vi "GenerateWaveform.vi"(5 "FPGA Cycle Parameters XY":T4={"FPGA Cycle Parameters X"={"Imaging cycles"=285714, "Settling cycles"=71429, "Resting cycles"=42857, "Phase advance per cycle"=0.0001399517059326172, "Imaging Multiplier advance per cycle"=0.00286865234375, "Settling Multiplier advance per cycle"=-0.0057373046875, "Imaging Initial Multiplier"=0.0, "Initial Phase"=0.0}, "FPGA Cycle Parameters Y"={"Imaging cycles"=285714, "Settling cycles"=71429, "Resting cycles"=42857, "Phase advance per cycle"=0.0001399517059326172, "Imaging Multiplier advance per cycle"=0.00286865234375, "Settling Multiplier advance per cycle"=-0.0057373046875, "Imaging Initial Multiplier"=0.0, "Initial Phase"=0.0}}, 6 "FPGA Cycle Counters XY In":T2, 7 "FPGA Scan Counters In":T1 {"Current part of waveform" items=["Imaging", "Settling", "Resting"]}) -> (0 "In Range":bool, 1 "Waveform Out":cluster{"Coerced Out":u16, "Coerced Out":u16}, 2 "FPGA Cycle Counters XY Out":T2, 3 "FPGA Scan Counters Out":T1 {"Current part of waveform" items=["Imaging", "Settling", "Resting"]})   [LabVIEW 2010]
uses:
  FPGA_Typedefs/FPGA Cycle Parameters XY.ctl
  FPGA_Typedefs/FPGA Cycle Parameters.ctl
  FPGA_Typedefs/FPGA Cycle Counters XY.ctl
  FPGA_Typedefs/FPGA Cycle Counters.ctl
  FPGA_Typedefs/FPGA Scan Counters.ctl
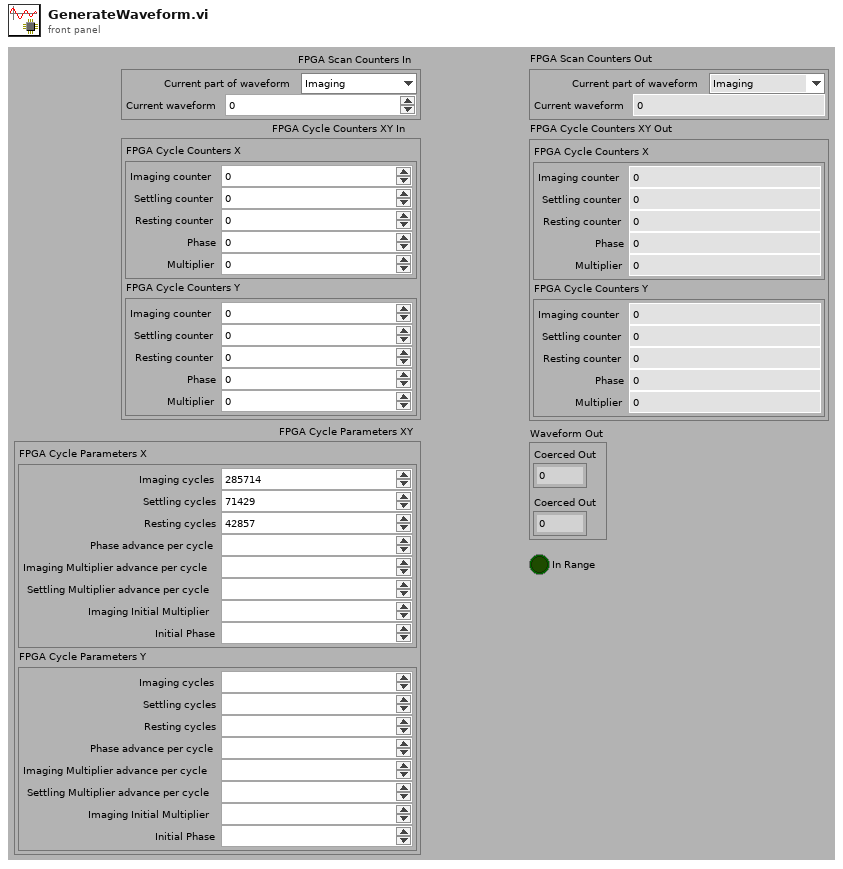
[diagram p1: front panel]
types:
  T1 = typedef "FPGA Scan Counters.ctl" = cluster{"Current part of waveform":u8, "Current waveform":u16}
  T2 = typedef "FPGA Cycle Counters XY.ctl" = cluster{"FPGA Cycle Counters X":T3, "FPGA Cycle Counters Y":T3}
  T3 = typedef "FPGA Cycle Counters.ctl" = cluster{"Imaging counter":i32, "Settling counter":i32, "Resting counter":i32, "Phase":fxp<+,32,1>, "Multiplier":fxp<+/-,43,12>}
  T4 = typedef "FPGA Cycle Parameters XY.ctl" = cluster{"FPGA Cycle Parameters X":T5, "FPGA Cycle Parameters Y":T5}
  T5 = typedef "FPGA Cycle Parameters.ctl" = cluster{"Imaging cycles":i32, "Settling cycles":i32, "Resting cycles":i32, "Phase advance per cycle":fxp<+,32,0>, "Imaging Multiplier advance per cycle":fxp<+/-,32,0>, "Settling Multiplier advance per cycle":fxp<+/-,32,0>, "Imaging Initial Multiplier":fxp<+/-,43,12>, "Initial Phase":fxp<+,32,1>}
  T6 = cluster{"Coerced U16 Out":u16, "Coerced U16 Out":u16}
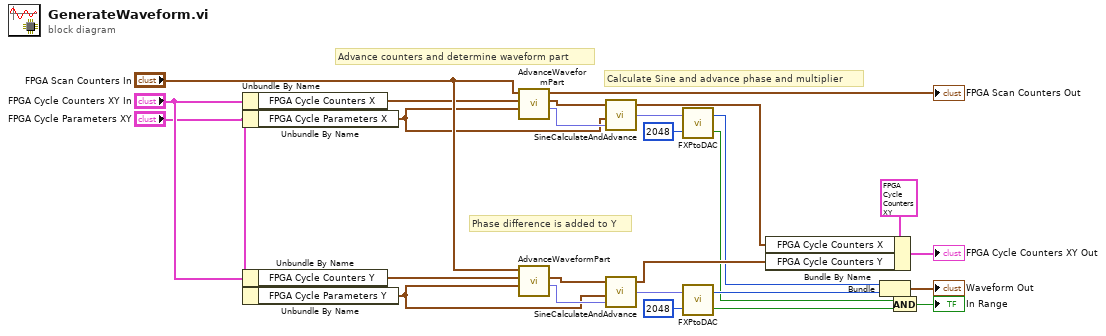
[diagram p0: block diagram]
diagram:
  # "Phase difference is added to Y"
  # "Calculate Sine and advance phase and multiplier"
  # "Advance counters and determine waveform part"
  n1 = Unbundle By Name("FPGA Cycle Counters XY In") -> ("FPGA Cycle Counters X"=w19:T3)
  n2 = Unbundle By Name("FPGA Cycle Parameters XY") -> ("FPGA Cycle Parameters X"=w4:T5)
  n3 = Unbundle By Name("FPGA Cycle Counters XY In") -> ("FPGA Cycle Counters Y"=w18:T3)
  n4 = Unbundle By Name("FPGA Cycle Parameters XY") -> ("FPGA Cycle Parameters Y"=w3:T5)
  n5 = call "AdvanceWaveformPart.vi"("FPGA Cycle Parameters"=w4, "FPGA Cycle Counters In"=w19, "FPGA Scan Counters In"="FPGA Scan Counters In") -> ("Multiplier advance per cycle"=w15:fxp<+/-,32,0>, "FPGA Cycle Counters Out"=w16:T3, "FPGA Scan Counters Out"=→"FPGA Scan Counters Out":T1)  [unwired: 3 in]
  n6 = call "AdvanceWaveformPart.vi"("FPGA Cycle Parameters"=w3, "FPGA Cycle Counters In"=w18, "FPGA Scan Counters In"="FPGA Scan Counters In") -> ("Multiplier advance per cycle"=w14:fxp<+/-,32,0>, "FPGA Cycle Counters Out"=w13:T3)  [unwired: 3 in, 1 out]
  n7 = call "SineCalculateAndAdvance.vi"("Multiplier advance per cycle"=w15, "FPGA Cycle Parameters In"=w4, "FPGA Cycle Counters In"=w16) -> ("Ramped sine"=w12:fxp<+/-,16,12>, "FPGA Cycle Counters Out"=w21:T3)  [unwired: 1 in]
  n8 = call "SineCalculateAndAdvance.vi"("Multiplier advance per cycle"=w14, "FPGA Cycle Parameters In"=w3, "FPGA Cycle Counters In"=w13) -> ("Ramped sine"=w11:fxp<+/-,16,12>, "FPGA Cycle Counters Out"=w20:T3)  [unwired: 1 in]
  n9 = call "FXPtoDAC.vi"("Offset"=i16 2048, "FXP In"=w12) -> ("In Range?"=w7:bool, "Coerced U16 Out"=w10:u16)
  n10 = call "FXPtoDAC.vi"("Offset"=i16 2048, "FXP In"=w11) -> ("In Range?"=w6:bool, "Coerced U16 Out"=w9:u16)
  n11 = Bundle By Name(cluster=T2 {"FPGA Cycle Counters X"={"Imaging counter"=0, "Settling counter"=0, "Resting counter"=0, "Phase"=0.0, "Multiplier"=0.0}, "FPGA Cycle Counters Y"={"Imaging counter"=0, "Settling counter"=0, "Resting counter"=0, "Phase"=0.0, "Multiplier"=0.0}} ("FPGA Waveform Counters Out"), "FPGA Cycle Counters X"=w21, "FPGA Cycle Counters Y"=w20) -> (→"FPGA Cycle Counters XY Out":T2)
  n12 = Bundle("Coerced U16 Out"=w10, "Coerced U16 Out"=w9) -> (→"Waveform Out":T6)  [unwired: 1 in]
  n13 = And(x=w7, y=w6) -> (x .and. y?=→"In Range":bool)
